vi "Run SV process.vi"(8 "error in (no error)":errorcluster, 11 "SV Data":T1={"Status notifier"=refnum, "Write FIFO ref"=refnum, "Read FIFO ref"=refnum, "Update Rate"=1, "Write Refs by Type"={"DBL Write"=[], "Bool Write"=[], "DBLIndex"=[], "BoolIndex"=[]}, "Read Refs by Type"={"DBL Read"=[], "Bool Read"=[], "DBLIndex"=[], "BoolIndex"=[]}, "WriteSize"=0, "ReadSize"=0}) -> (0 "error out":errorcluster, 3 "SV Data":T1={"Status notifier"=refnum, "Write FIFO ref"=refnum, "Read FIFO ref"=refnum, "Update Rate"=1, "Write Refs by Type"={"DBL Write"=[], "Bool Write"=[], "DBLIndex"=[], "BoolIndex"=[]}, "Read Refs by Type"={"DBL Read"=[], "Bool Read"=[], "DBLIndex"=[], "BoolIndex"=[]}, "WriteSize"=0, "ReadSize"=0})   [LabVIEW 2017, in "Shared Variable Interface.lvlib"]
uses:
  Shared Variable Interface.lvlib
  DataTypes/DBL/ReadSV.vi
  DataTypes/Bool/ReadSV.vi
  DataTypes/DBL/WriteSV.vi
  DataTypes/Bool/WriteSV.vi
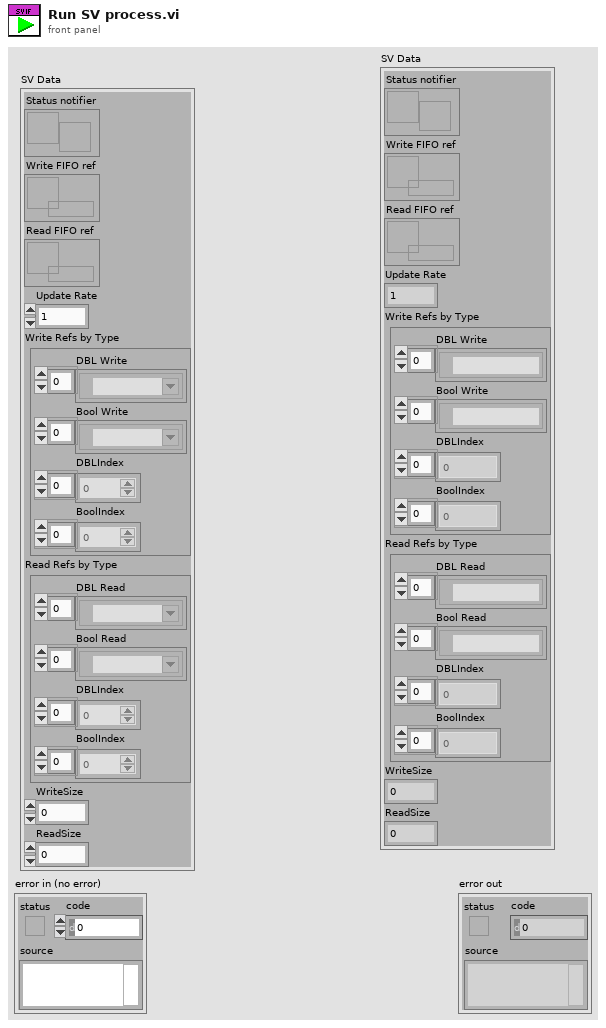
[diagram p1: front panel]
types:
  T1 = cluster{"Status notifier":refnum<notifier>, "Write FIFO ref":refnum<k33>, "Read FIFO ref":refnum<k33>, "Update Rate":u32, "Write Refs by Type":cluster{"DBL Write":refnum<k21>[], "Bool Write":refnum<k21>[], "DBLIndex":i32[], "BoolIndex":i32[]}, "Read Refs by Type":cluster{"DBL Read":refnum<k21>[], "Bool Read":refnum<k21>[], "DBLIndex":i32[], "BoolIndex":i32[]}, "WriteSize":i32, "ReadSize":i32}
  T2 = cluster{"DBL Write":refnum<k21>[], "Bool Write":refnum<k21>[], "DBLIndex":i32[], "BoolIndex":i32[]}
  T3 = cluster{"DBL Read":refnum<k21>[], "Bool Read":refnum<k21>[], "DBLIndex":i32[], "BoolIndex":i32[]}
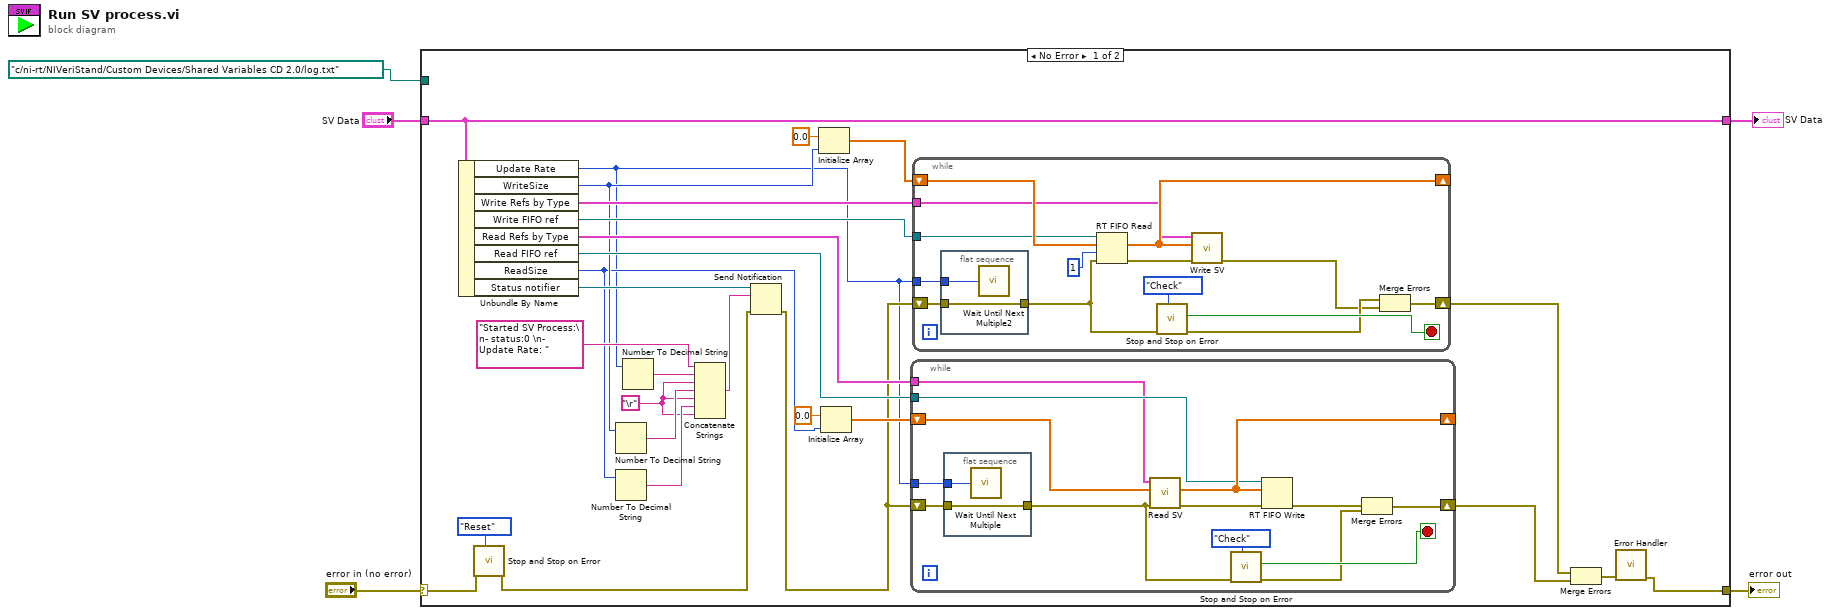
[diagram p0: block diagram]
diagram:
  n1 = case shown="No Error" "error in (no error)" {
    selector: "error in (no error)" -> [w25 w65]
    tunnel: [w26 w65] -> w4
    tunnel: path "c:/ni-rt/NIVeriStand/Custom Devices/Shared Variables CD 2.0/log.txt" ("Path to Trace Log") -> [_ _]
    tunnel: "SV Data" -> [w10 w64]
    tunnel: [w10 w64] -> w1
    frame No Error {
      w13 = "\r" ("string")
      n2 = Unbundle By Name(w10) -> ("Update Rate"=w6:u32, "WriteSize"=w8:i32, "Write Refs by Type"=w20:T2, "Write FIFO ref"=w32:refnum<k33>, "Read Refs by Type"=w21:T3, "Read FIFO ref"=w22:refnum<k33>, "ReadSize"=w7:i32, "Status notifier"=w9:refnum<notifier>)
      n3 = call "Stop and Stop on Error.vi"("Action"=enum16{"Check", "Reset"}."Reset", "error in (no error)"=w25) -> ("error out"=w12:errorcluster)  [unwired: 8 in, 1 out]
      n4 = Number To Decimal String(number=w8) -> (decimal integer string=w15:string)  [unwired: 1 in]
      n5 = Number To Decimal String(number=w7) -> (decimal integer string=w14:string)  [unwired: 1 in]
      n6 = Number To Decimal String(number=w6) -> (decimal integer string=w23:string)  [unwired: 1 in]
      n7 = Concatenate Strings("Started SV Process:\n- status:0 \n- Update Rate: " ("notification"), w23, w13, w15, w13, w14, w13) -> (w24:string)
      n8 = Send Notification(notification=w24, notifier=w9, error in (no error)=w12) -> (error out=w11:errorcluster)  [unwired: 1 out]
      n9 = Initialize Array(0.0 ("element"), w8) -> (w18:dbl[])
      n10 = Initialize Array(0.0 ("element"), w7) -> (w16:dbl[])
      n11 = while {
        tunnel: w22 -> [w53]
        shift-right: [w55] -> w30
        shift-left: w11 -> [w50]
        tunnel: w6 -> [w49]
        tunnel: w21 -> [w52]
        shift-right: [w58] -> _
        shift-left: w16 -> [w57]
        stop <- w60 stop-if-true
        n12 = flat-sequence {
          tunnel: w50 -> [w63]
          tunnel: [w63] -> w51
          tunnel: w49 -> [w62]
          frame #0 {
            n13 = call "Wait Until Next Multiple"("Count(uSec)"=w62) -> ()  [unwired: 1 out]
          }
        }
        n14 = call "Read SV.vi"("error in (no error)"=w51, "Data"=w57, "Read Refs by Type"=w52) -> ("error out"=w56:errorcluster, "Data Out"=w58:dbl[])  [unwired: 7 in]
        n15 = call "Stop and Stop on Error.vi"("Action"=enum16{"Check", "Reset"}."Check", "error in (no error)"=w51) -> ("error out"=w59:errorcluster, "Stop?"=w60:bool)  [unwired: 8 in]
        n16 = RT FIFO Write(0:w53, 1:w58, 3:w56) -> (11:w54:errorcluster)  [unwired: 2 in, 3 out]
        n17 = Merge Errors(w54, w59) -> (w55:errorcluster)
      }
      n18 = while {
        tunnel: w32 -> [w33]
        shift-right: [w36] -> w31
        shift-left: w11 -> [w44]
        tunnel: w6 -> [w43]
        tunnel: w20 -> [w34]
        shift-right: [w40] -> _
        shift-left: w18 -> [w41]
        stop <- w46 stop-if-true
        n19 = flat-sequence {
          tunnel: w44 -> [w48]
          tunnel: [w48] -> w35
          tunnel: w43 -> [w47]
          frame #0 {
            n20 = call "Wait Until Next Multiple2"("Count(uSec)"=w47) -> ()  [unwired: 1 out]
          }
        }
        n21 = RT FIFO Read(0:w33, 1:w41, 2:1 ("timeout in ms (0)"), 3:w35) -> (9:w40:dbl[], 11:w39:errorcluster)  [unwired: 3 out]
        n22 = call "Stop and Stop on Error.vi"("Action"=enum16{"Check", "Reset"}."Check", "error in (no error)"=w35) -> ("error out"=w38:errorcluster, "Stop?"=w46:bool)  [unwired: 8 in]
        n23 = call "Write SV.vi"("error in (no error)"=w39, "Data"=w40, "Write Refs by Type"=w34) -> ("error out"=w37:errorcluster)  [unwired: 8 in]
        n24 = Merge Errors(w38, w37) -> (w36:errorcluster)
      }
      n25 = Merge Errors(w31, w30) -> (w27:errorcluster)
      n26 = call "Error Handler.vi"("error in (no error)"=w27) -> ("error out"=w26:errorcluster)  [unwired: 10 in]
    }
    frame Error {
    }
  }
  "error out" <- w4
  "SV Data" <- w1
